vi "Create Menus.vi"(6 "menu options":cluster{"open":bool, "save":bool, "view":bool}={"open"=TRUE, "save"=FALSE, "view"=FALSE}, 8 "error in (no error)":errorcluster, 11 "Application Data in":T1) -> (0 "error out":errorcluster, 3 "Application Data out":T1)   [LabVIEW 2017, in "DSF Core.lvlib"]
uses:
  DSF Core.lvlib
  Application Data.ctl
  <vilib>/NI/Memory Manager/Classes/Pointer/Pointer.lvclass
  Classes/Framework/Framework.lvclass
  Buffer Reader/Buffer Data.ctl
  Classes/Buffer/Buffer.lvclass
  Classes/Transfer Group Status/Status.lvclass
  Typedefs/DSF Engine Framework Configuration.ctl
  Typedefs/DSF Engine Plugin Configuration.ctl
  Typedefs/DSF Timing Info.ctl
  Typedefs/DSF Engine Plugin Thread Configuration.ctl
  Typedefs/DSF Settings Info.ctl
  Typedefs/DSF Engine Transfer Group Configuration.ctl
  Typedefs/DSF Direction.ctl
  Typedefs/DSF Engine Transfer Configuration.ctl
  Typedefs/DSF Byte Order.ctl
  Typedefs/DSF Engine Channel Configuration.ctl
  Typedefs/DSF Data Type.ctl
  Typedefs/DSF Timeout Behavior.ctl
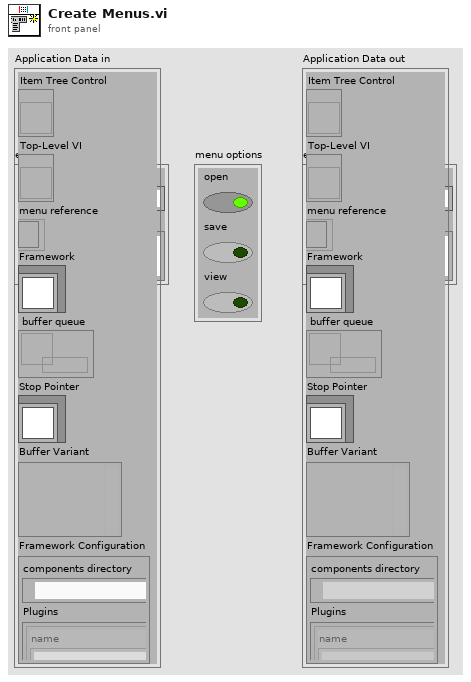
[diagram p1: front panel]
types:
  T1 = typedef "DSF Core.lvlib/Application Data.ctl" = cluster{"Item Tree Control":refnum<vi>, "Top-Level VI":refnum<vi>, "menu reference":refnum<k9>, "Framework":refnum<class "Framework.lvclass">, "buffer queue":refnum<queue>, "Stop Pointer":refnum<class "Pointer.lvclass">, "Buffer Variant":variant, "Framework Configuration":T2}
  T2 = typedef "DSF Core.lvlib/DSF Engine Framework Configuration.ctl" = cluster{"components directory":path, "Plugins":T3[]}
  T3 = typedef "DSF Core.lvlib/DSF Engine Plugin Configuration.ctl" = cluster{"name":string, "components":string[], "cycle timing":T4, "threads":T5[], "Transfer Groups":T7[], "settings":T6}
  T4 = typedef "DSF Core.lvlib/DSF Timing Info.ctl" = cluster{"priority":u64, "decimation":u64, "offset":u64}
  T5 = typedef "DSF Core.lvlib/DSF Engine Plugin Thread Configuration.ctl" = cluster{"buffer converter settings":T6, "transceiver settings":T6, "processor":i32, "priority offset":i16}
  T6 = typedef "DSF Core.lvlib/DSF Settings Info.ctl" = cluster{"key":string, "value":string}[]
  T7 = typedef "DSF Core.lvlib/DSF Engine Transfer Group Configuration.ctl" = cluster{"name":string, "direction":T8, "cycle timing":T4, "thread index":i32, "settings":T6, "Transfers":T9[], "timeout behavior":T13}
  T8 = typedef "DSF Core.lvlib/DSF Direction.ctl" = enum8{"Tx", "Rx"}
  T9 = typedef "DSF Core.lvlib/DSF Engine Transfer Configuration.ctl" = cluster{"name":string, "byte order":T10, "settings":T6, "channels":T11[]}
  T10 = typedef "DSF Core.lvlib/DSF Byte Order.ctl" = enum8{"big-endian", "little-endian"}
  T11 = typedef "DSF Core.lvlib/DSF Engine Channel Configuration.ctl" = cluster{"string offset":u64, "string data type":T12, "engine data type":T12, "name":string, "settings":T6}
  T12 = typedef "DSF Core.lvlib/DSF Data Type.ctl" = enum8{"Bool", "SGL", "DBL", "I8", "I16", "I32", "I64", "U8", "U16", "U32", "U64"}
  T13 = typedef "DSF Core.lvlib/DSF Timeout Behavior.ctl" = enum8{"Increment Late Count", "Throw Error"}
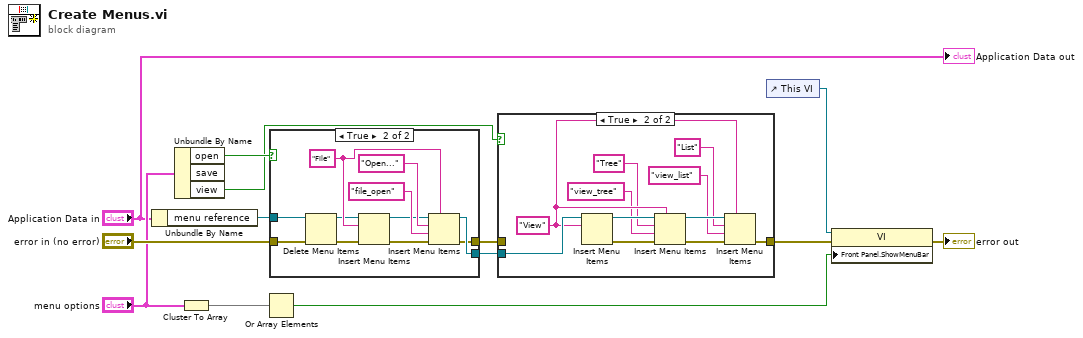
[diagram p0: block diagram]
diagram:
  n1 = Unbundle By Name("Application Data in") -> ("menu reference"=w1:refnum<k9>)
  n2 = Unbundle By Name("menu options") -> ("open"=w11:bool, "view"=w10:bool)  [unwired: 1 out]
  n3 = Cluster To Array(cluster="menu options") -> (array=w7:bool[])
  n4 = Or Array Elements(Boolean array=w7) -> (logical OR=w5:bool)
  n5 = case shown="True" w11 {
    tunnel: "error in (no error)" -> [w14 w26]
    tunnel: [w15 w24] -> w12
    tunnel: w1 -> [w15 w17]
    tunnel: [w14 w16] -> w9
    frame False {
    }
    frame True {
      w21 = "File" ("item names")
      n6 = Delete Menu Items(6:w26, 9:w17) -> (0:w25:errorcluster, 3:w18:refnum<k9>)  [unwired: 2 in]
      n7 = Insert Menu Items(6:w25, 8:w21, 9:w18) -> (0:w19:errorcluster, 3:w20:refnum<k9>)  [unwired: 3 in, 1 out]
      n8 = Insert Menu Items(5:w21, 6:w19, 7:"file_open" ("item tags"), 8:"Open..." ("item names"), 9:w20) -> (0:w16:errorcluster, 3:w24:refnum<k9>)  [unwired: 1 in, 1 out]
    }
  }
  n9 = case shown="True" w10 {
    tunnel: [w27 w38] -> w4
    tunnel: w12 -> [_ w37]
    tunnel: w9 -> [w27 _]
    frame False {
    }
    frame True {
      w35 = "View" ("item names")
      n10 = Insert Menu Items(8:w35, 9:w37) -> (0:w31:errorcluster, 3:w30:refnum<k9>)  [unwired: 4 in, 1 out]
      n11 = Insert Menu Items(5:w35, 6:w31, 7:"view_tree" ("item tags"), 8:"Tree" ("item names"), 9:w30) -> (0:w36:errorcluster, 3:w34:refnum<k9>)  [unwired: 1 in, 1 out]
      n12 = Insert Menu Items(5:w35, 6:w36, 7:"view_list" ("item tags"), 8:"List" ("item names"), 9:w34) -> (0:w38:errorcluster)  [unwired: 1 in, 2 out]
    }
  }
  n13 = control-ref of="This VI"() -> (w6:refnum<vi>)
  n14 = property class="VI"(reference=w6, error in=w4, "Front Panel.ShowMenuBar"=w5) -> (error out=→"error out":errorcluster)  [unwired: 1 out]
  "Application Data out" <- "Application Data in"
